vi "LoadConfig_AxisSpace.vi"(8 "error in (no error)":errorcluster, 11 "Path (.AxisSpace.cfg)":path) -> (0 "error out":errorcluster, 1 "file or folder exists?":bool, 2 "Axis Space":T1 {"Axis" items=["Axis 1"=1, "Axis 2"=2, "Axis 3"=3, "Axis 4"=4, "Axis 5"=5, "Axis 6"=6, "Axis 7"=7, "Axis 8"=8]})   [LabVIEW 2010]
doc: "Loads axis space config from file."
uses:
  Typedefs/AxisSpaceCfg_ArrayofAxisCfg.ctl
  Typedefs/AxisCfg_cluster.ctl
  <vilib>/Motion/FlexMotion/CustomControls/CustomControls.llb/Axis To Read.flx
  <vilib>/Utility/xml.llb/Read From XML File(string).vi
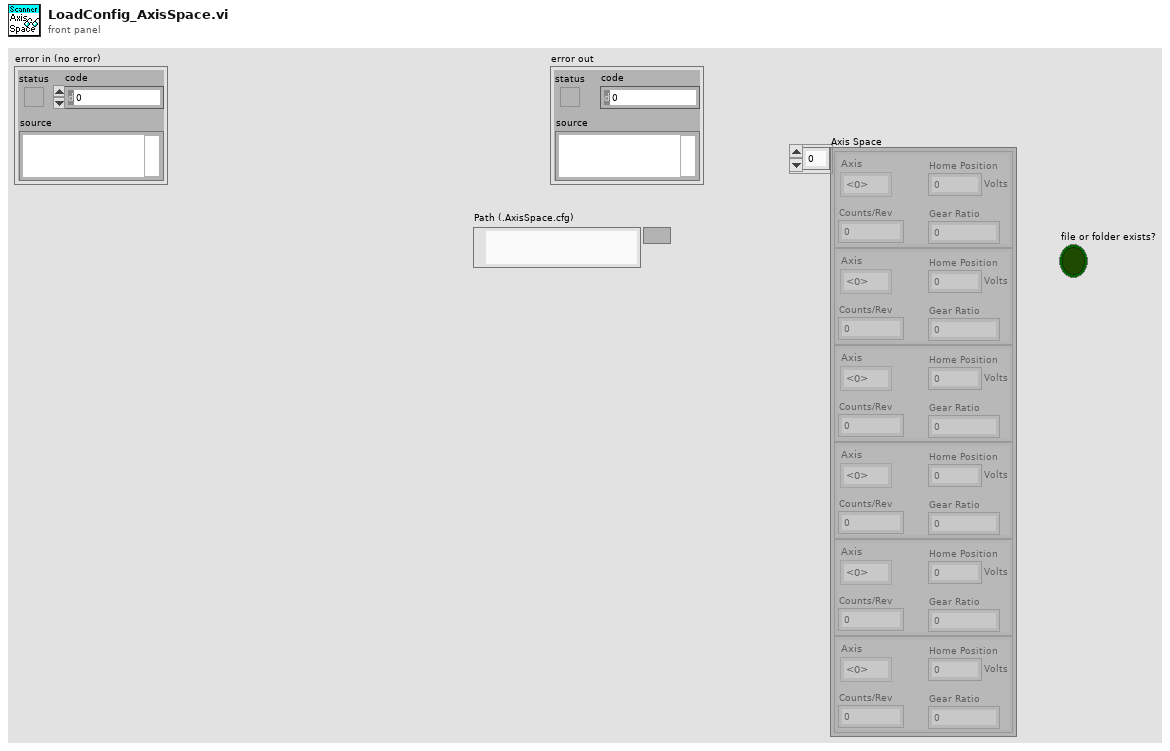
[diagram p1: front panel]
types:
  T1 = typedef "AxisSpaceCfg_ArrayofAxisCfg.ctl" = T2[]
  T2 = typedef "AxisCfg_cluster.ctl" = cluster{"Axis":T3, "Counts/Rev":dbl, "Gear Ratio":dbl, "Home Position":dbl}
  T3 = typedef "Axis To Read.flx" = u16
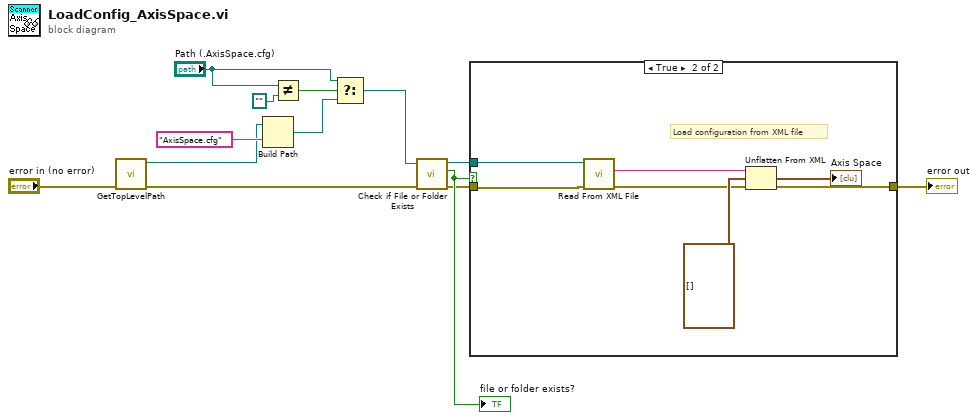
[diagram p0: block diagram]
diagram:
  n1 = call "GetTopLevelPath.vi"("error in"="error in (no error)") -> ("error out"=w2:errorcluster, "path"=w1:path)  [unwired: 9 in]
  n2 = Build Path(base path=w1, name or relative path="AxisSpace.cfg") -> (appended path=w7:path)
  n3 = Not Equal?(x="Path (.AxisSpace.cfg)", y=path "") -> (x != y?=w9:bool)
  n4 = Select(t="Path (.AxisSpace.cfg)", s=w9, f=w7) -> (s? t:f=w6:path)
  n5 = call <vilib>:"Check if File or Folder Exists.vi"("error in (no error)"=w2, "path"=w6) -> ("error out"=w5:errorcluster, "file or folder exists?"=w12:bool, "dup path"=w13:path)  [unwired: 7 in]
  "file or folder exists?" <- w12
  n6 = case shown="True" w12 {
    tunnel: w13 -> [_ w19]
    tunnel: w5 -> [w14 w17]
    tunnel: [w14 w15] -> w4
    frame False {
    }
    frame True {
      # "Load configuration from XML file"
      n7 = call-poly <vilib>:"Read From XML File.vi"("error in (no error)"=w17, "XML File Path"=w19) -> ("error out"=w16:errorcluster, "XML Elements"=w21:string)  [unwired: 7 in, 1 out]
      n8 = Unflatten From XML(xml string=w21, type=T1 [] ("Axis Space"), error in (no error)=w16) -> (value=→"Axis Space":T1, error out=w15:errorcluster)
    }
  }
  "error out" <- w4
